vi "insertSpace.vi"(4 "deltaY":u16, 6 "deltaX":u16, 8 "error in (no error)":errorcluster, 10 "origin":T1, 11 "AbstractDiagram In":refnum<class "AbstractDiagram.lvclass">) -> (0 "error out":errorcluster, 3 "AbstractDiagram Out":refnum<class "AbstractDiagram.lvclass">)   [LabVIEW 2023, in "TLC_Scripto.lvlib" / "AbstractDiagram.lvclass"]
uses:
  AbstractDiagram.lvclass
  Ctrls/point.ctl
  Read GObjects.vi
  GObject/GObject.lvclass
  TLC_Scripto.lvlib
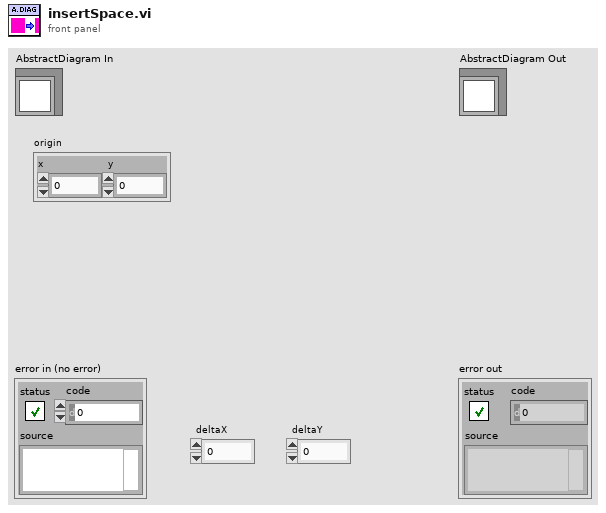
[diagram p1: front panel]
types:
  T1 = typedef "TLC_Scripto.lvlib/point.ctl" = cluster{"x":i32, "y":i32}
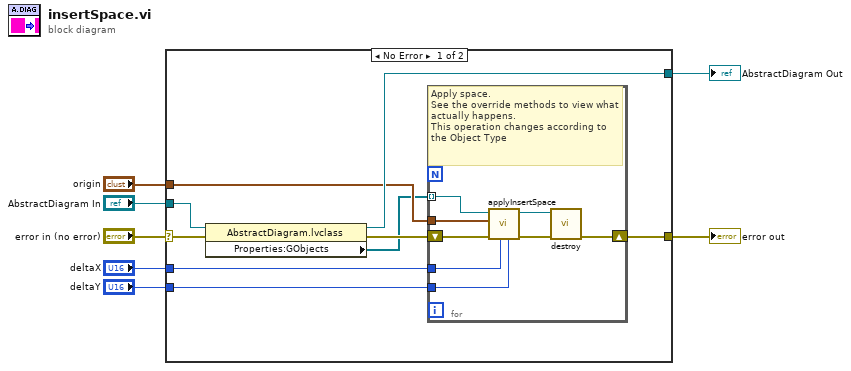
[diagram p0: block diagram]
diagram:
  n1 = case shown="No Error" "error in (no error)" {
    selector: "error in (no error)" -> [w15 w26]
    tunnel: [w10 w26] -> w6
    tunnel: [w14 w25] -> w4
    tunnel: "AbstractDiagram In" -> [w13 w25]
    tunnel: "origin" -> [w9 _]
    tunnel: "deltaX" -> [w12 _]
    tunnel: "deltaY" -> [w11 _]
    frame No Error {
      n2 = property class="AbstractDiagram.lvclass"(reference=w13, error in=w15) -> (reference out=w14:refnum<class "AbstractDiagram.lvclass">, error out=w16:errorcluster, "Properties:GObjects"=w8:refnum<class "GObject.lvclass">[])
      n3 = for {
        tunnel: w8 -> [w22] mode=indexing
        shift-right: [w20] -> w10
        shift-left: w16 -> [w24]
        tunnel: w12 -> [w17]
        tunnel: w11 -> [w18]
        tunnel: w9 -> [w21]
        # "Apply space.\nSee the override methods to view what actually happens.\nThis operation changes according to the Object Type"
        n4 = call "applyInsertSpace.vi"("deltaY"=w18, "deltaX"=w17, "error in (no error)"=w24, "origin"=w21, "GObject in"=w22) -> ("error out"=w23:errorcluster, "GObject out"=w19:refnum<class "GObject.lvclass">)  [unwired: 5 in]
        n5 = call-dynamic "destroy.vi"("Error In"=w23, "Generic In"=w19) -> ("Error Out"=w20:errorcluster)  [unwired: 9 in]
      }
    }
    frame Error {
    }
  }
  "error out" <- w6
  "AbstractDiagram Out" <- w4
